vi "PostCopyScripting.vi"(10 "MetaDataObj":refnum<class "MetaDataObj.lvclass">, 11 "User Project":refnum<vi>) -> ()   [LabVIEW 2013, in "editorscriptingobject.lvclass"]
uses:
  editorscriptingobject.lvclass
  <resource>/dialog/NewProjectWizard/MetaDataObj/MetaDataObj.lvclass
  editorscriptingobject.lvclass/editorscriptingobject.ctl
  Read library name.vi
  <vilib>/Utility/EditLVLibs/Edit LVLibs.lvlib
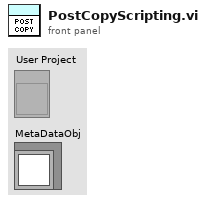
[diagram p1: front panel]
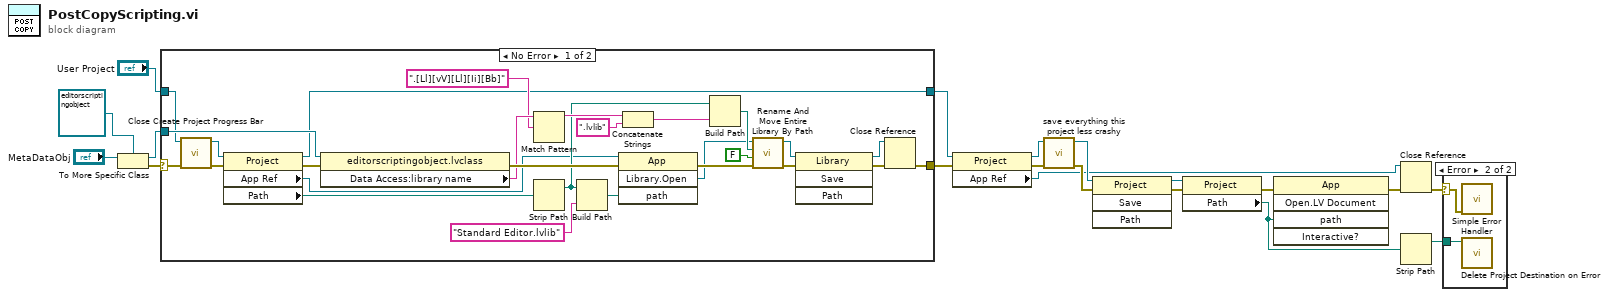
[diagram p0: block diagram]
diagram:
  n1 = To More Specific Class(target class=refnum<class "editorscriptingobject.lvclass"> refnum ("DecideProjectFeatures.lvclass"), reference="MetaDataObj") -> (specific class reference=w10:refnum<class "editorscriptingobject.lvclass">, error out=w17:errorcluster)  [unwired: 1 in]
  n2 = case shown="No Error" w17 {
    selector: w17 -> [w43 w47]
    tunnel: [w20 w48] -> w7
    tunnel: "User Project" -> [w42 w48]
    tunnel: [w21 w47] -> w6
    tunnel: w10 -> [w44 _]
    frame No Error {
      n3 = call <resource>:"Close Create Project Progress Bar.vi"("error in (no error)"=w43, "Project"=w42) -> ("error out"=w40:errorcluster, "dup Project"=w41:refnum<vi>)  [unwired: 8 in]
      n4 = property class="Project"(reference=w41, error in=w40) -> (reference out=w20:refnum<vi>, error out=w46:errorcluster, "App Ref"=w30:refnum<vi>, "Path"=w45:path)
      n5 = property class="editorscriptingobject.lvclass"(reference=w44, error in=w46) -> (error out=w38:errorcluster, "Data Access:library name"=w37:string)  [unwired: 1 out]
      n6 = Match Pattern(string=w37, regular expression=".[Ll][vV][Ll][Ii][Bb]") -> (before substring=w35:string)  [unwired: 1 in, 3 out]
      n7 = Strip Path(path=w45) -> (stripped path=w32:path)  [unwired: 1 out]
      n8 = Build Path(base path=w32, name or relative path="Standard Editor.lvlib") -> (appended path=w29:path)
      n9 = invoke class="App" method="Library.Open"(reference=w30, error in=w38, "path"=w29) -> (error out=w31:errorcluster, "Open Library"=w27:refnum<vi>)  [unwired: 1 in, 2 out]
      n10 = Concatenate Strings(w35, ".lvlib" ("string")) -> (w33:string)
      n11 = Build Path(base path=w32, name or relative path=w33) -> (appended path=w28:path)
      n12 = call <vilib>:"Rename And Move Entire Library By Path.vi"("error in (no error)"=w31, "Delete old directory if empty after move? (T)"=FALSE, "New library path"=w28, "Library ref in"=w27) -> ("error out"=w25:errorcluster, "Library ref out"=w24:refnum<vi>)  [unwired: 6 in]
      n13 = invoke class="Library" method="Save"(reference=w24, error in=w25) -> (reference out=w22:refnum<vi>, error out=w23:errorcluster)  [unwired: 2 in, 2 out]
      n14 = Close Reference(reference=w22, error in (no error)=w23) -> (error out=w21:errorcluster)
    }
    frame Error {
    }
  }
  n15 = property class="Project"(reference=w7, error in=w6) -> (reference out=w4:refnum<vi>, error out=w5:errorcluster, "App Ref"=w3:refnum<vi>)
  n16 = call "save everything this project less crashy.vi"("error in"=w5, "Project in"=w4) -> ("error out"=w9:errorcluster, "Project out"=w8:refnum<vi>)  [unwired: 8 in]
  n17 = invoke class="Project" method="Save"(reference=w8, error in=w9) -> (reference out=w13:refnum<vi>, error out=w14:errorcluster)  [unwired: 2 in, 2 out]
  n18 = property class="Project"(reference=w13, error in=w14) -> (error out=w16:errorcluster, "Path"=w11:path)  [unwired: 1 out]
  n19 = invoke class="App" method="Open.LV Document"(error in=w16, "path"=w11) -> (error out=w15:errorcluster)  [unwired: 3 in, 4 out]
  n20 = Close Reference(reference=w3, error in (no error)=w15) -> (error out=w2:errorcluster)
  n21 = Strip Path(path=w11) -> (stripped path=w1:path)  [unwired: 1 out]
  n22 = case shown="Error" w2 {
    selector: w2 -> [_ w49]
    tunnel: w1 -> [_ w50]
    frame No Error {
    }
    frame Error {
      n23 = call <vilib>:"Simple Error Handler.vi"("error in (no error)"=w49) -> ()  [unwired: 4 in, 5 out]
      n24 = call <resource>:"Delete Project Destination on Error.vi"("Project Destination Root"=w50) -> ()  [unwired: 11 in]
    }
  }
